vi "Min-Max.vi"(0 "VISA resource name":refnum<visa-resource-name>, 7 "Channel (1)":i32=1 min=1 max=16 step=1, 11 "error in (no error)":errorcluster) -> (4 "VISA resource name out":refnum<visa-resource-name>, 6 "Max Value":dbl min=0.0 max=63200000.0 step=1e-05 format="%^.5e", 10 "Min Value":dbl min=0.0 max=63200000.0 step=1e-05 format="%^.5e", 15 "error out":errorcluster)   [LabVIEW 2012, in "Lake Shore Cryotronics 370.lvlib"]
doc: "This VI querys the instrument for a channel's min/max readings."
uses:
  <instrlib>/Lake Shore Cryotronics 370/Lake Shore Cryotronics 370.lvlib
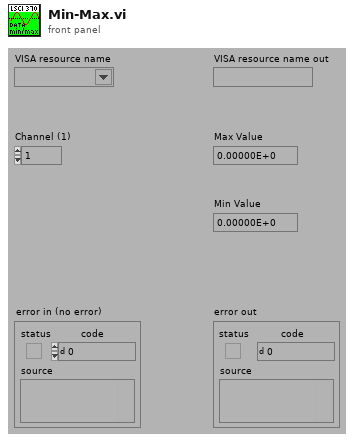
[diagram p1: front panel]
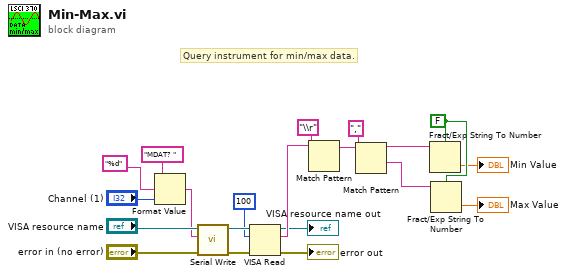
[diagram p0: block diagram]
diagram:
  w8 = FALSE ("use system decimal point (T)")
  # "Query instrument for min/max data."
  n1 = Format Value(string ("")="MDAT? ", format string="%d", value (0)="Channel (1)") -> (output string=w3:string)
  n2 = call <instrlib>:"Serial Write.vi"("error in (no error)"="error in (no error)", "Write Buffer (\"\")"=w3, "VISA resource name"="VISA resource name") -> ("error out"=w19:errorcluster, "VISA resource name out"=w20:refnum<visa-resource-name>)  [unwired: 6 in, 1 out]
  n3 = VISA Read(VISA resource name=w20, byte count=100, error in (no error)=w19) -> (VISA resource name out=→"VISA resource name out":refnum<visa-resource-name>, read buffer=w17:string, error out=→"error out":errorcluster)  [unwired: 1 out]
  n4 = Match Pattern(string=w17, regular expression="\\r") -> (before substring=w14:string)  [unwired: 1 in, 3 out]
  n5 = Match Pattern(string=w14, regular expression=",") -> (before substring=w13:string, after substring=w12:string)  [unwired: 1 in, 2 out]
  n6 = Fract/Exp String To Number(use system decimal point (T)=w8, string=w13) -> (number=→"Min Value":dbl)  [unwired: 2 in, 1 out]
  n7 = Fract/Exp String To Number(use system decimal point (T)=w8, string=w12) -> (number=→"Max Value":dbl)  [unwired: 2 in, 1 out]
